vi "XY Graph Remove Data Point.vi"(8 "Error In":errorcluster, 9 "Excluded Plots":i32[](array[numeric]), 10 "Coords":T1, 11 "XYGraph in":refnum<vi>) -> (0 "Error Out":errorcluster, 1 "Point  Index":i32, 2 "Distance to Plot":dbl, 3 "Plot Number":i32, 4 "Message":string, 6 "Removed?":bool)   [LabVIEW 2021, in "XY Graph Add-Ons.lvlib"]
uses:
  XY Graph Add-Ons.lvlib
  <vilib>/Utility/miscctls.llb/LVPoint32TypeDef.ctl
  XY Graph Selected Plot Info.ctl
  XY Graph Refnum.ctl
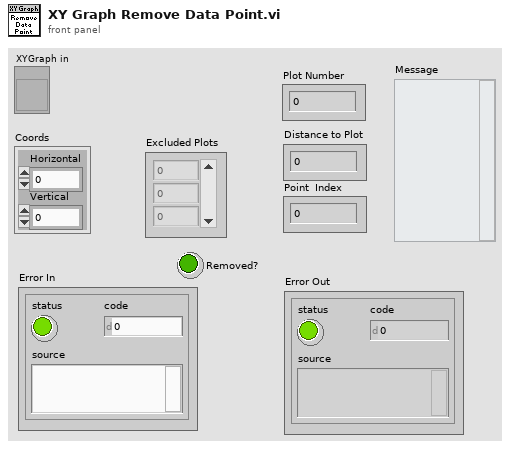
[diagram p1: front panel]
types:
  T1 = typedef "LVPoint32TypeDef.ctl" = cluster{"Horizontal":i32, "Vertical":i32}
  T2 = typedef "XY Graph Add-Ons.lvlib/XY Graph Selected Plot Info.ctl" = cluster{"Multiplot XY Graph":T3, "Mouse Coordinates":T1, "Plot Index":i32}
  T3 = typedef "XY Graph Add-Ons.lvlib/XY Graph Refnum.ctl" = refnum<vi>
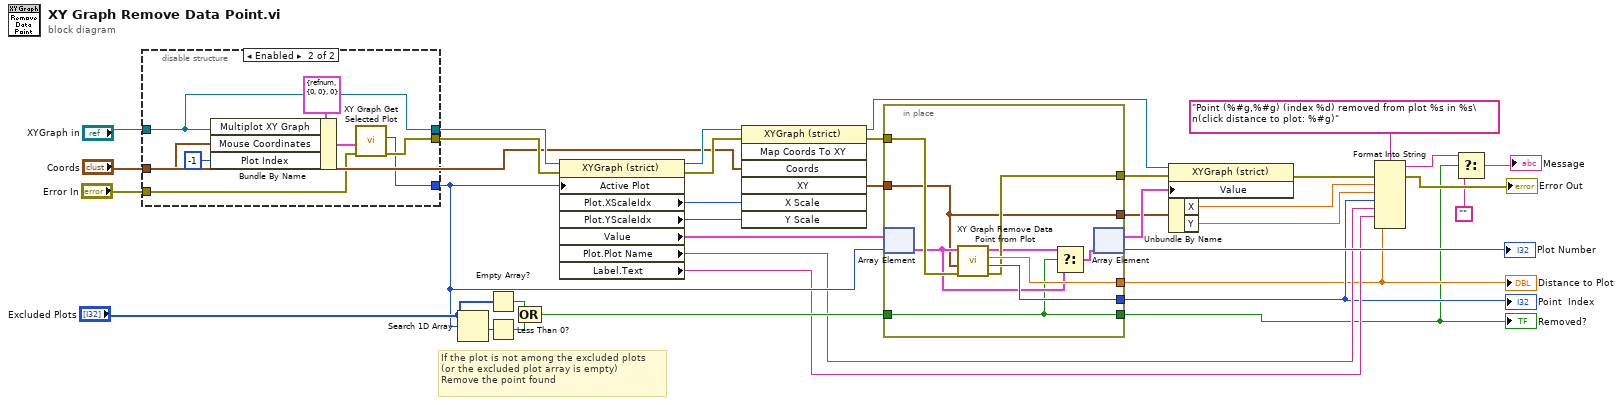
[diagram p0: block diagram]
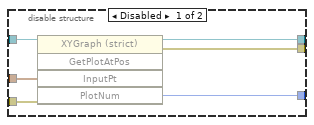
[diagram p2: hidden frame]
diagram:
  # "If the plot is not among the excluded plots\n(or the excluded plot array is empty)\nRemove the point found"
  n1 = disable-structure shown="Enabled" {
    disable-tunnel: "XYGraph in" -> [w42 w44]
    disable-tunnel: [w41 w44] -> w35
    disable-tunnel: [w40 w45] -> w34
    disable-tunnel: "Error In" -> [w39 w46]
    disable-tunnel: [w38 w43] -> w15
    disable-tunnel: "Coords" -> [w37 w48]
    frame Disabled {
      n2 = invoke class="XYGraph (strict)" method="GetPlotAtPos"(reference=w42, error in=w39, "InputPt"=w37) -> (reference out=w41:refnum<vi>, error out=w40:errorcluster, "PlotNum"=w38:i32)  [unwired: 2 in, 2 out]
    }
    frame Enabled {
      n3 = Bundle By Name(cluster=T2 {"Multiplot XY Graph"=refnum, "Mouse Coordinates"={"Horizontal"=0, "Vertical"=0}, "Plot Index"=0} ("Selected Plot Info"), "Multiplot XY Graph"=w44, "Mouse Coordinates"=w48, "Plot Index"=-1) -> (w49:T2)
      n4 = call "XY Graph Get Selected Plot.vi"("error in (no error)"=w46, "Selected Plot Info"=w49) -> ("error out"=w45:errorcluster, "Plot Index"=w43:i32)  [unwired: 4 in, 4 out]
    }
  }
  n5 = Search 1D Array(1D array="Excluded Plots", element=w15) -> (index of element=w22:i32)  [unwired: 1 in]
  n6 = Empty Array?(array="Excluded Plots") -> (empty?=w20:bool)
  n7 = Less Than 0?(x=w22) -> (x < 0?=w19:bool)
  n8 = Compound Arithmetic op=OR(w20, w19) -> (w14:bool)
  n9 = property class="XYGraph (strict)"(reference=w35, error in=w34, "Active Plot"=w15) -> (reference out=w32:refnum<vi>, error out=w31:errorcluster, "Plot.XScaleIdx"=w30:u32, "Plot.YScaleIdx"=w29:u32, "Value"=w28:cluster{"X Array":dbl[], "Y Array":dbl[]}[], "Plot.Plot Name"=w8:string, "Label.Text"=w7:string)
  n10 = invoke class="XYGraph (strict)" method="Map Coords To XY"(reference=w32, error in=w31, "Coords"="Coords", "X Scale"=w30, "Y Scale"=w29) -> (reference out=w27:refnum<vi>, error out=w24:errorcluster, "XY"=w25:cluster{"X":dbl, "Y":dbl})  [unwired: 2 in, 4 out]
  n11 = in-place {
    in-place-border: w25 -> [w51]
    in-place-border: [w59] -> w6
    in-place-border: [w58] -> w5
    in-place-border: w24 -> [w57]
    in-place-border: [w56] -> w23
    in-place-border: w14 -> [w52]
    in-place-border: [w52] -> w2
    in-place-border: [w51] -> w13
    n12 = in-place-array #1(w28, w15) -> (w54:cluster{"X Array":dbl[], "Y Array":dbl[]})
    n13 = call "XY Graph Remove Data Point from Plot.vi"("Error In"=w57, "Point"=w51, "Plot in"=w54) -> ("Error Out"=w56:errorcluster, "Point  Index"=w59:i32, "Distance to Plot"=w58:dbl, "Plot out"=w55:cluster{"X Array":dbl[], "Y Array":dbl[]})  [unwired: 5 in]
    n14 = Select(t=w55, s=w52, f=w54) -> (s? t:f=w53:cluster{"X Array":dbl[], "Y Array":dbl[]})
    n15 = in-place-array #1(w53) -> (w26:cluster{"X Array":dbl[], "Y Array":dbl[]}[], →"Plot Number":i32)
  }
  "Distance to Plot" <- w5
  "Point  Index" <- w6
  "Removed?" <- w2
  n16 = property class="XYGraph (strict)"(reference=w27, error in=w23, "Value"=w26) -> (error out=w17:errorcluster)  [unwired: 1 out]
  n17 = Unbundle By Name(w13) -> ("X"=w10:dbl, "Y"=w9:dbl)
  n18 = Format Into String(format string="Point (%#g,%#g) (index %d) removed from plot %s in %s\n(click distance to plot: %#g)", error in=w17, w10, w9, w6, w8, w7, w5) -> (resulting string=w4:string, error out=→"Error Out":errorcluster)  [unwired: 1 in]
  n19 = Select(t=w4, s=w2, f="") -> (s? t:f=→"Message":string)
